vi "Muted.vi"(7 "Direction":T1, 8 "error in (no error)":errorcluster, 10 "Index":i32, 11 "VoiceMeeterRemote in":refnum<class "VoiceMeeterRemote.lvclass">) -> (0 "error out":errorcluster, 1 "Muted?":bool, 3 "VoiceMeeterRemote out":refnum<class "VoiceMeeterRemote.lvclass">)   [LabVIEW 2022 SP3, in "VoiceMeeterRemote.lvlib" / "VoiceMeeterRemote.lvclass"]
doc: "Returns whether the specified input or output index is currently muted."
uses:
  VoiceMeeterRemote.lvclass
  Direction.ctl
  VoiceMeeterRemote.lvlib
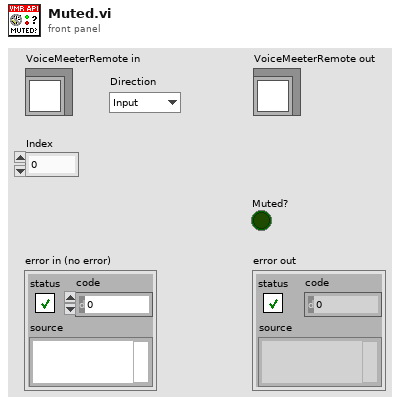
[diagram p1: front panel]
types:
  T1 = typedef "VoiceMeeterRemote.lvlib/Direction.ctl" = enum16{"Input", "Output"}
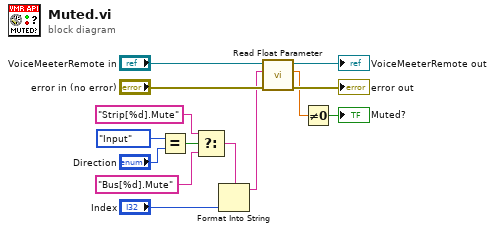
[diagram p0: block diagram]
diagram:
  n1 = Equal?(x=Direction."Input", y="Direction") -> (x = y?=w12:bool)
  n2 = Select(t="Strip[%d].Mute", s=w12, f="Bus[%d].Mute") -> (s? t:f=w9:string)
  n3 = Format Into String(format string=w9, "Index") -> (resulting string=w3:string)  [unwired: 2 in, 1 out]
  n4 = call "Read Float Parameter.vi"("error in (no error)"="error in (no error)", "Parameter Name"=w3, "VoiceMeeterRemote in"="VoiceMeeterRemote in") -> ("error out"=→"error out":errorcluster, "Value"=w2:sgl, "VoiceMeeterRemote out"=→"VoiceMeeterRemote out":refnum<class "VoiceMeeterRemote.lvclass">)  [unwired: 6 in]
  n5 = Not Equal To 0?(x=w2) -> (x != 0?=→"Muted?":bool)
